vi "Main.vi"() -> ()   [LabVIEW 2016]
uses:
  <vilib>/picture/picture.llb/imagedata.ctl
panel:
  in  "Path":path
  in  "pConvertInfo In 2":T1
  out "QuitFlag":bool
  in  "image data":T2 caption="图像数据"
  in  "Rectangle":T3
  in  "pConvertInfo In":T1
  out "Picture":picture
  out "Acquired Frames/s":dbl
  out "Processed Frames/s":dbl
  in  "SavePic":bool
  in  "TriggerSource":u16(ring) items=["Software", "Line1", "Line2"]
  in  "ExecuteSoftTrig":bool
  in  "CloseTrig":bool
  in  "OpenTrig":bool
  in  "Stop":bool
  in  "Play":bool
  in  "Quit":bool
  in  "handle":i64
  in  "Height":i64
  in  "Width":i64
  in  "ExposureAuto":u16(ring) items=["Off", "Once", "Continuous"]
  in  "PixelFormat":u16(ring) items=["BayerRG8", "BayerGB8", "BayerRG10", "BayerGB10", "BayerRG10Packed", "BayerGB10Packed"]
  in  "GainRaw":dbl
  in  "ExposureTime":dbl
  in  "Close":bool
  in  "Open":bool
  out "IsGrabbing":bool
  out "HasDevices":bool
  out "TrigModeOn":bool
  in  "DeviceOpened":bool
  in  "DeviceList":u16(ring)
  out "error out":errorcluster
  in  "Discovery":bool
  in  "error in":errorcluster
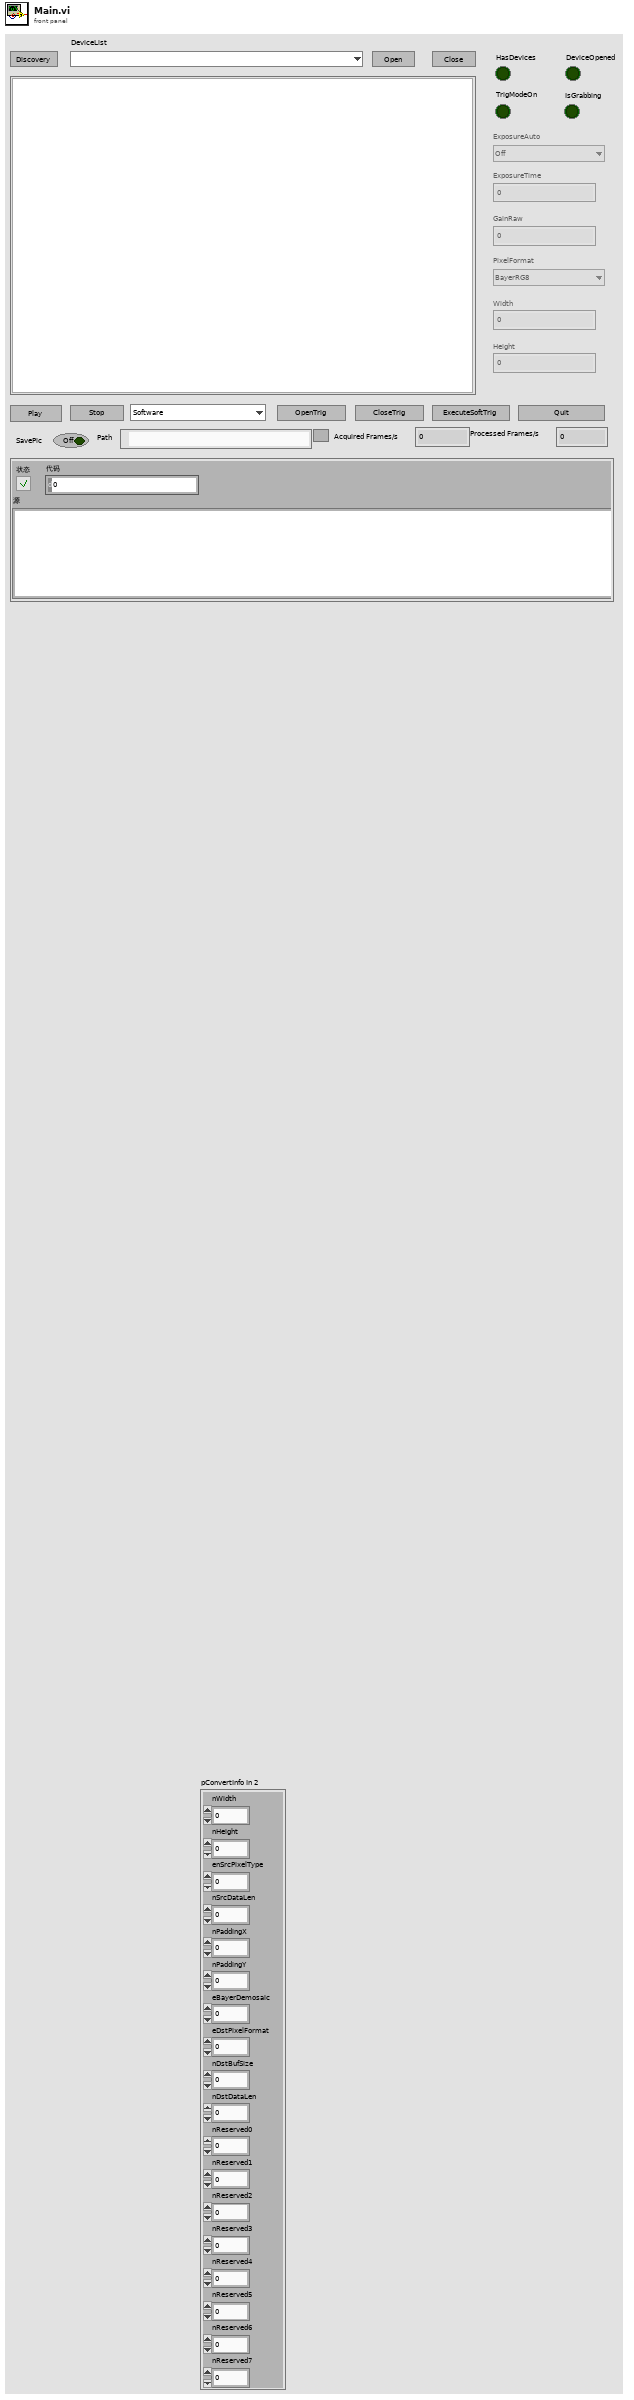
[diagram p1: front panel]
types:
  T1 = cluster{"nWidth":u32, "nHeight":u32, "enSrcPixelType":u32, "nSrcDataLen":u32, "nPaddingX":u32, "nPaddingY":u32, "eBayerDemosaic":u32, "eDstPixelFormat":u32, "nDstBufSize":u32, "nDstDataLen":u32, "nReserved0":u32, "nReserved1":u32, "nReserved2":u32, "nReserved3":u32, "nReserved4":u32, "nReserved5":u32, "nReserved6":u32, "nReserved7":u32}
  T2 = typedef "imagedata.ctl" = cluster{"image type":i32, "image depth":i32, "image":u8[], "mask":u8[], "colors":u32[], "Rectangle":cluster{"left":i16, "top":i16, "right":i16, "bottom":i16}}
  T3 = cluster{"left":i16, "top":i16, "right":i16, "bottom":i16}
  T4 = enum8{"Enabled", "Disabled", "Disabled and Grayed Out"}
  T5 = cluster{"blockId":u64, "status":u32, "width":u32, "height":u32, "size":u32, "pixelFormat":u32, "timeStamp":u64, "chunkCount":u32, "paddingX":u32, "paddingY":u32, "recvFrameTime":u32}
  T6 = cluster{"blockId":u64, "status":u32, "width":u32, "height":u32, "size":u32, "pixelFormat":i32, "timeStamp":u64, "chunkCount":u32, "paddingX":u32, "paddingY":u32, "recvFrameTime":u32}
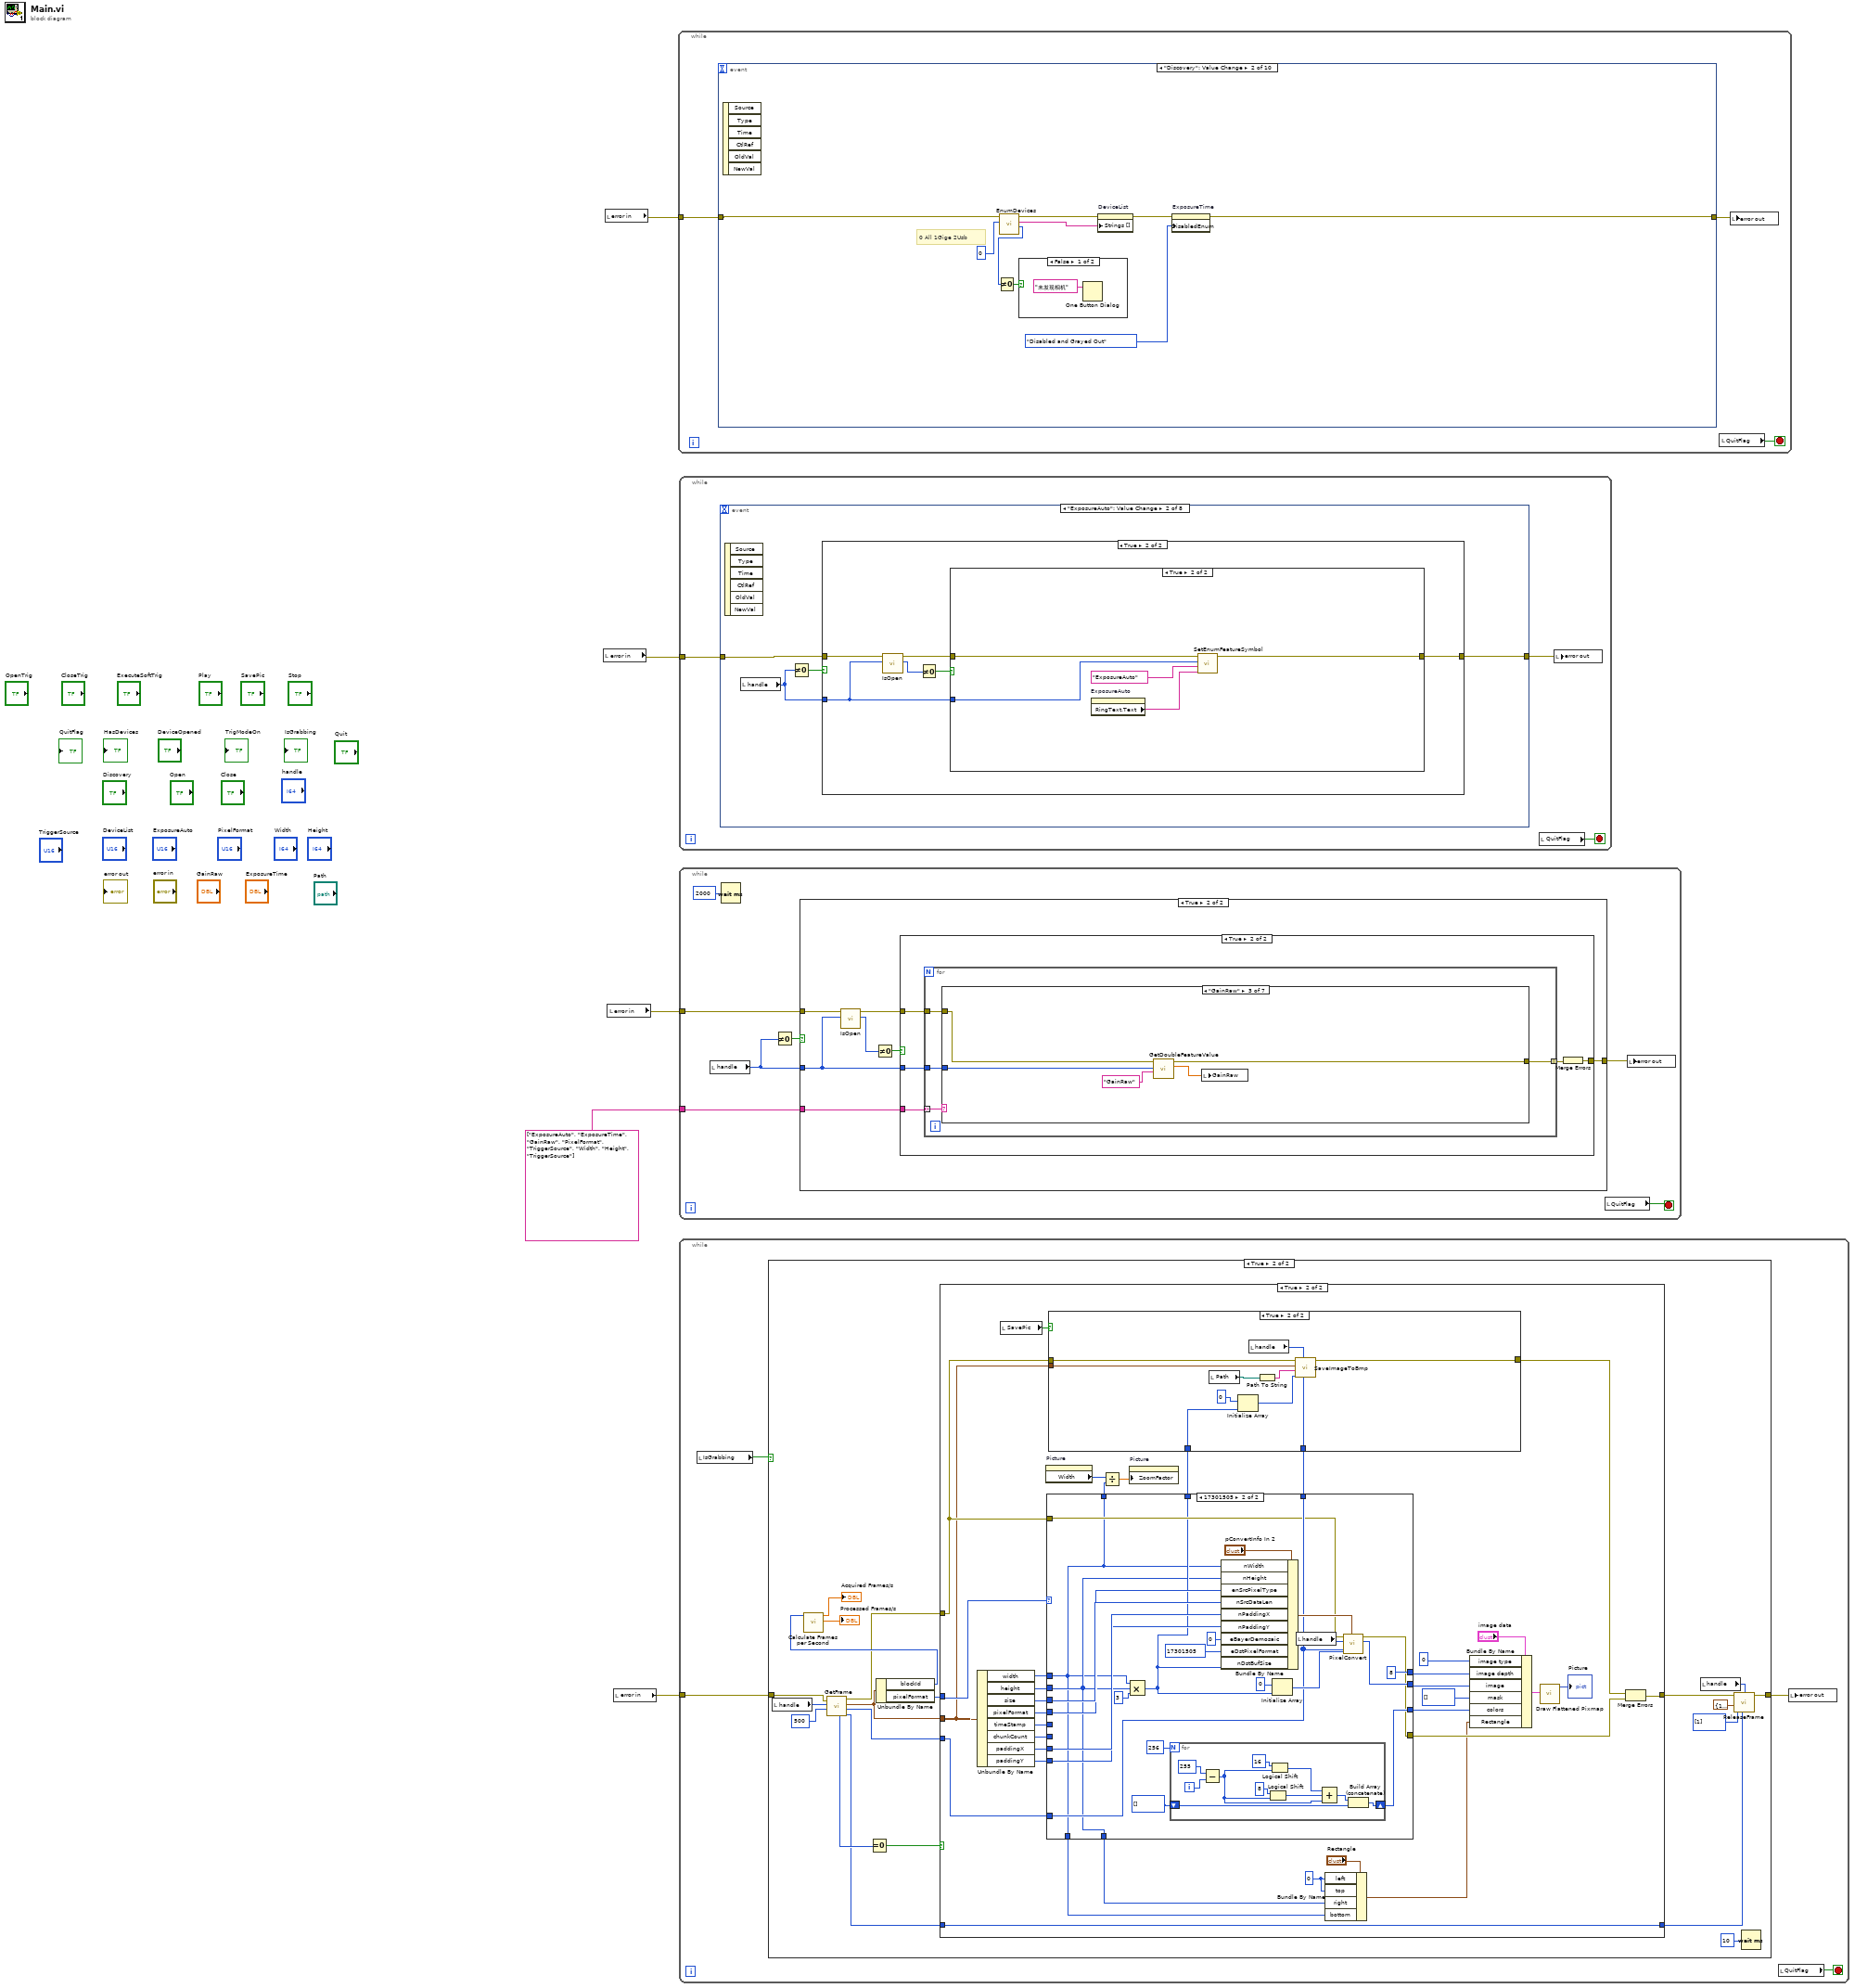
[diagram p0: block diagram]
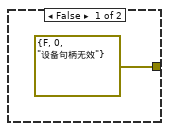
[diagram p2: hidden frame]
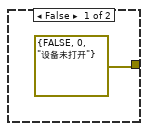
[diagram p3: hidden frame]
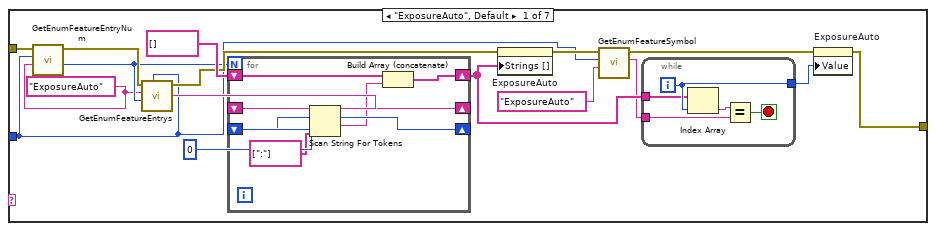
[diagram p4: hidden frame]
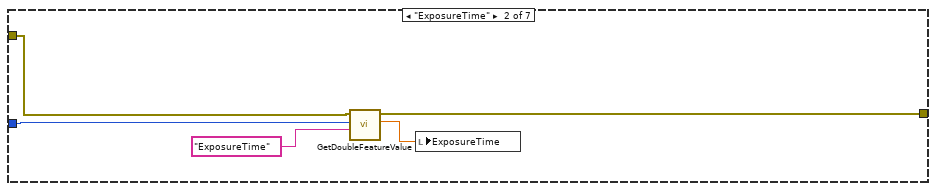
[diagram p5: hidden frame]
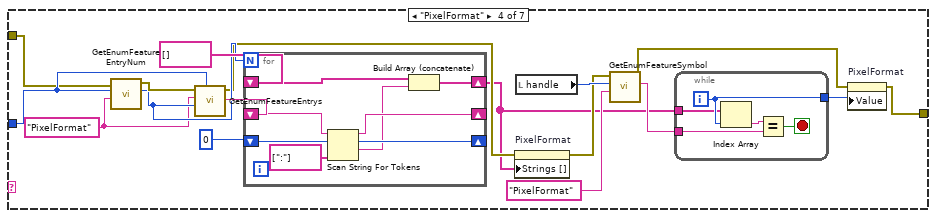
[diagram p6: hidden frame]
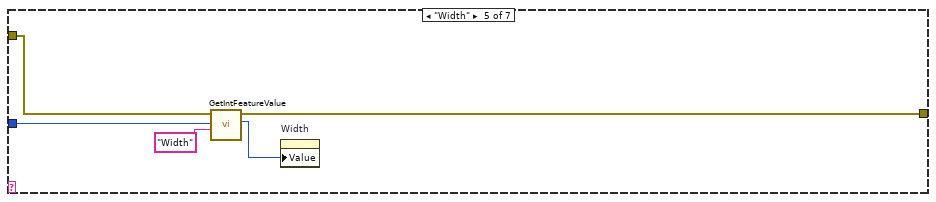
[diagram p7: hidden frame]
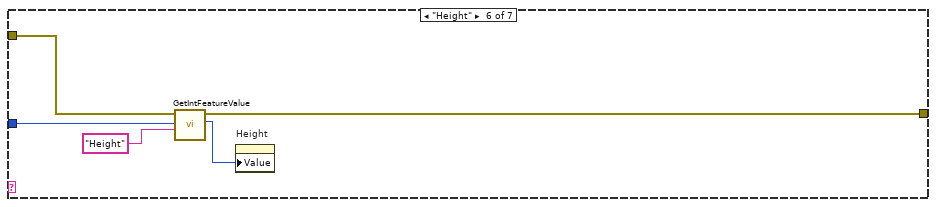
[diagram p8: hidden frame]
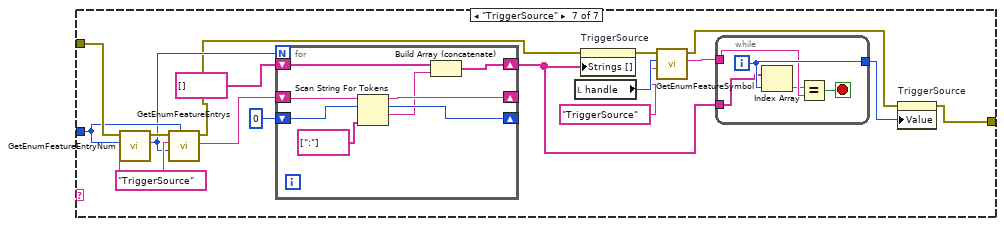
[diagram p9: hidden frame]
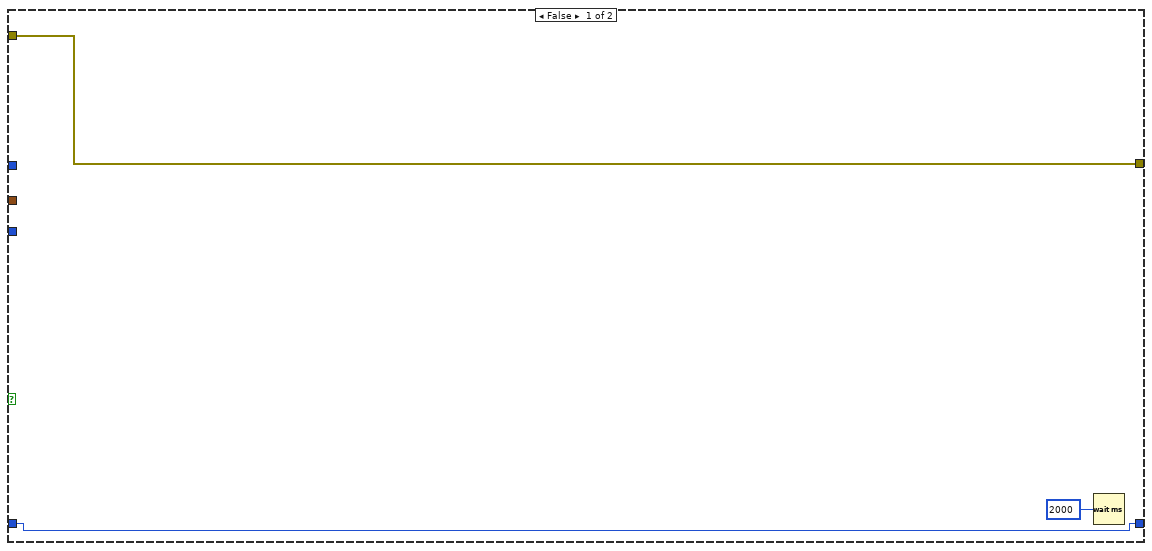
[diagram p11: hidden frame]
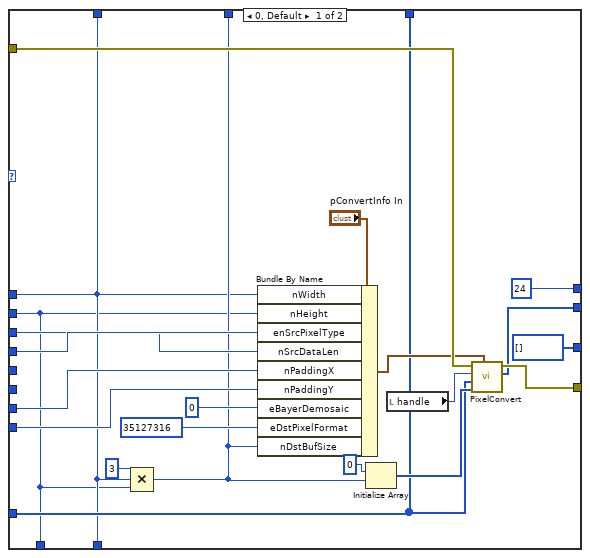
[diagram p13: hidden frame]
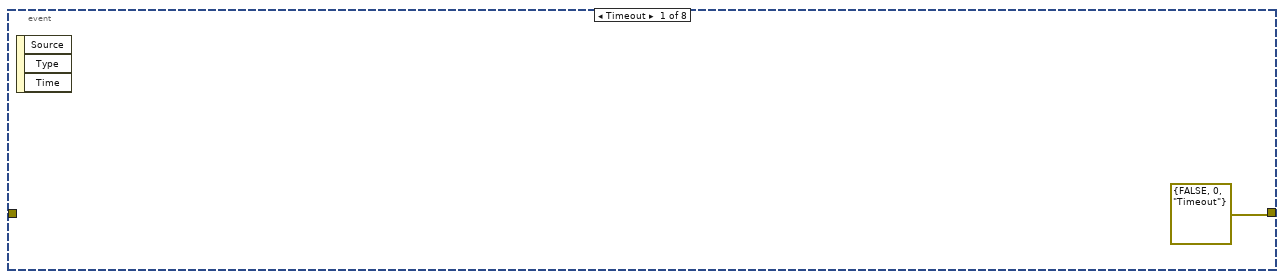
[diagram p14: hidden frame]
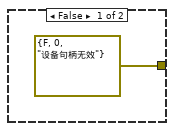
[diagram p15: hidden frame]
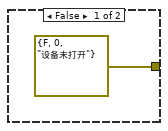
[diagram p16: hidden frame]
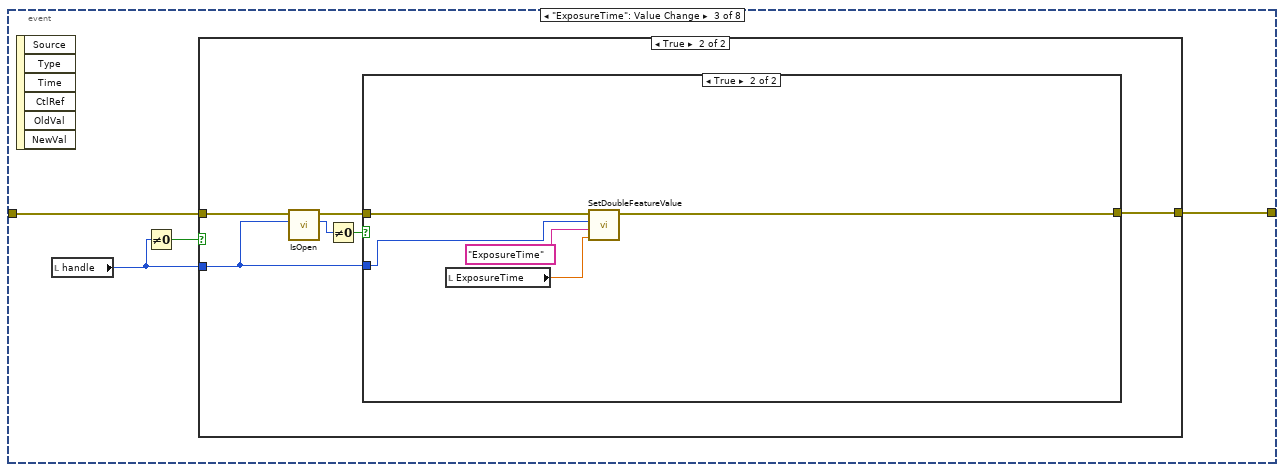
[diagram p17: hidden frame]
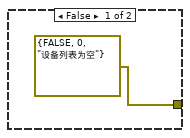
[diagram p18: hidden frame]
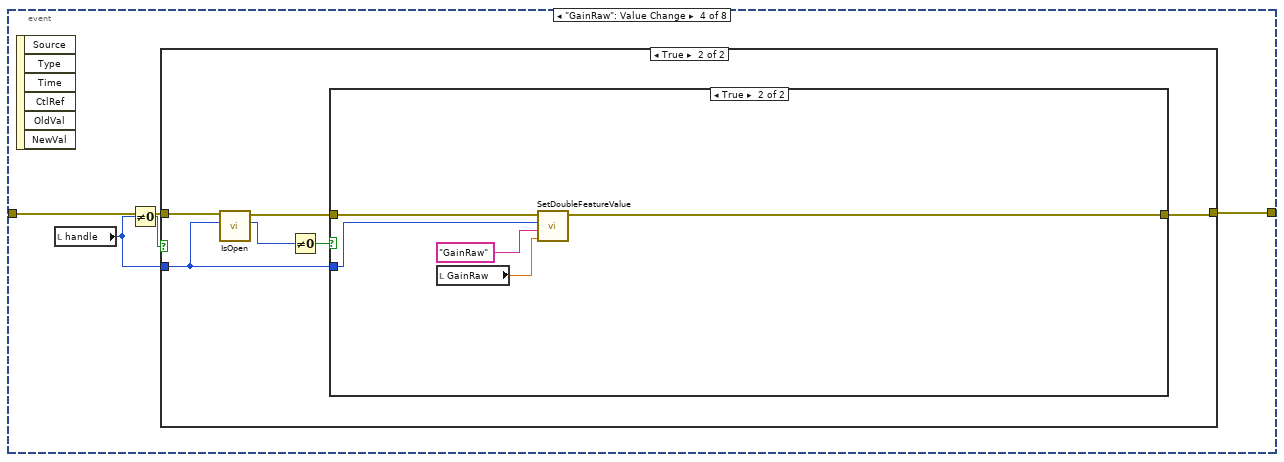
[diagram p20: hidden frame]
diagram:
  n1 = local read "error in"() -> (w4:errorcluster)
  n2 = local read "error in"() -> (w5:errorcluster)
  n3 = local read "error in"() -> (w2:errorcluster)
  n4 = local read "error in"() -> (w1:errorcluster)
  n5 = while {
    tunnel: w5 -> [w8]
    stop <- w7 stop-if-true
    n6 = event shown="[1] \"Discovery\": Value Change" {
      selector: _ -> [_ _ _ _ _ _ _ _ _ _]
      dyn-events: _ -> [_ _ _ _ _ _ _ _ _ _]
      timeout: _ -> [_ _ _ _ _ _ _ _ _ _]
      tunnel: w8 -> [_ w17 w23 w74 w87 w140 w147 w151 w169 w188]
      tunnel: [errorcluster {FALSE, 0, "Timeout"} w13 w22 w61 w85 w131 w143 w150 w155 w173] -> w6
      event Timeout {
        n7 = event-data() -> ()  [unwired: 1 in, 3 out]
      }
      event "Discovery": Value Change {
        # "0 All 1Gige 2Usb"
        n8 = event-data() -> ()  [unwired: 1 in, 6 out]
        n9 = call "EnumDevices.vi"("interfaceType"=u32 0, "error in"=w17) -> ("nDevNum"=w10:i32, "cameraKeyList"=w15:string[], "error out"=w16:errorcluster)  [unwired: 7 in]
        n10 = Not Equal To 0?(x=w10) -> (x != 0?=w11:bool)
        n11 = case shown="False" w11 {
          frame False {
            n12 = One Button Dialog(message="未发现相机") -> ()  [unwired: 1 in, 1 out]
          }
          frame True {
            n13 = local write "HasDevices"(TRUE ("HasDevices")) -> ()
          }
        }
        n14 = property on="DeviceList" class="Ring (strict)"(error in=w16, "Strings []"=w15) -> (error out=w12:errorcluster)  [unwired: 1 in, 1 out]
        n15 = property on="ExposureTime" class="DigNum (strict)"(error in=w12, "DisabledEnum"=T4."Disabled and Grayed Out" ("Disabled")) -> (error out=w13:errorcluster)  [unwired: 1 in, 1 out]
      }
      event "Quit": Value Change {
        n16 = event-data() -> ()  [unwired: 1 in, 6 out]
        n17 = flat-sequence {
          tunnel: w23 -> [w26]
          tunnel: [w26] -> w21
          tunnel: [w35] -> w22
          tunnel: w21 -> [w53]
          frame #0 {
            n18 = local write "SavePic"(FALSE ("SavePic")) -> ()
            n19 = Wait (ms)(milliseconds to wait=u32 500) -> ()  [unwired: 1 out]
          }
          frame #1 {
            (unwired) T4."Enabled" ("Disabled")
            (unwired) T4."Disabled and Grayed Out" ("Disabled")
            n20 = local read "handle"() -> (w29:i64)
            n21 = call "SetEnumFeatureSymbol.vi"("pEnumSymbol"="Off", "pFeatureName"="TriggerMode", "handle"=w29, "error in (no error)"=w53) -> ("return type"=w50:i32, "error out"=w48:errorcluster)  [unwired: 6 in]
            n22 = Equal To 0?(x=w50) -> (x = 0?=w49:bool)
            n23 = case shown="True" w49 {
              frame False {
              }
              frame True {
                n24 = local write "TrigModeOn"(FALSE ("IsGrabbing")) -> ()
              }
            }
            n25 = call "StopGrabbing.vi"("handle"=w29, "error in (no error)"=w48) -> ("return type"=w28:i32, "error out"=w36:errorcluster)  [unwired: 8 in]
            n26 = Equal To 0?(x=w28) -> (x = 0?=w27:bool)
            n27 = case shown="True" w27 {
              frame False {
              }
              frame True {
                n28 = local write "IsGrabbing"(FALSE ("IsGrabbing")) -> ()
              }
            }
            n29 = property on="ExposureAuto" class="Ring (strict)"(error in=w36, "DisabledEnum"=T4."Disabled and Grayed Out" ("Disabled")) -> (error out=w39:errorcluster)  [unwired: 1 in, 1 out]
            n30 = property on="GainRaw" class="DigNum (strict)"(error in=w39, "DisabledEnum"=T4."Disabled and Grayed Out" ("Disabled")) -> (error out=w37:errorcluster)  [unwired: 1 in, 1 out]
            n31 = property on="Height" class="DigNum (strict)"(error in=w37, "DisabledEnum"=T4."Disabled and Grayed Out" ("Disabled")) -> (error out=w45:errorcluster)  [unwired: 1 in, 1 out]
            n32 = property on="PixelFormat" class="Ring (strict)"(error in=w45, "DisabledEnum"=T4."Disabled and Grayed Out" ("Disabled")) -> (error out=w40:errorcluster)  [unwired: 1 in, 1 out]
            n33 = property on="ExposureTime" class="DigNum (strict)"(error in=w40, "DisabledEnum"=T4."Disabled and Grayed Out" ("Disabled")) -> (error out=w46:errorcluster)  [unwired: 1 in, 1 out]
            n34 = property on="Width" class="DigNum (strict)"(error in=w46, "DisabledEnum"=T4."Disabled and Grayed Out" ("Disabled")) -> (error out=w30:errorcluster)  [unwired: 1 in, 1 out]
            n35 = call "Close.vi"("handle"=w29, "error in (no error)"=w30) -> ("return type"=w33:i32, "error out"=w35:errorcluster)  [unwired: 8 in]
            n36 = Equal To 0?(x=w33) -> (x = 0?=w34:bool)
            n37 = case shown="True" w34 {
              frame False {
              }
              frame True {
                n38 = local write "DeviceOpened"(FALSE ("DeviceOpened")) -> ()
              }
            }
            n39 = local write "HasDevices"(FALSE ("HasDevices")) -> ()
            n40 = local write "QuitFlag"(FALSE) -> ()
            n41 = property on="DeviceList" class="Ring (strict)"("Strings []"=string[] []) -> ()  [unwired: 2 in, 2 out]
          }
        }
      }
      event "Open": Value Change {
        (unwired) T4."Enabled" ("Disabled")
        n42 = event-data() -> ()  [unwired: 1 in, 6 out]
        n43 = property on="DeviceList" class="Ring (strict)"(error in=w74) -> (error out=w76:errorcluster, "Value"=w75:u16)  [unwired: 1 in, 1 out]
        n44 = call "OpenDevice.vi"("pIdentifier"=w75, "error in (no error)"=w76) -> ("handle"=w60:i64, "retrun type"=w58:i32, "error out"=w62:errorcluster)  [unwired: 7 in]
        n45 = local write "handle"(w60) -> ()
        n46 = Equal To 0?(x=w58) -> (x = 0?=w59:bool)
        n47 = case shown="True" w59 {
          tunnel: w58 -> [w79 _]
          frame False {
            n48 = Number To Decimal String(number=w79) -> (decimal integer string=w78:string)  [unwired: 1 in]
            n49 = Concatenate Strings("打开相机失败" ("string"), w78) -> (w80:string)
            n50 = One Button Dialog(message=w80) -> ()  [unwired: 1 in, 1 out]
          }
          frame True {
            n51 = local write "DeviceOpened"(TRUE ("DeviceOpened")) -> ()
          }
        }
        n52 = property on="ExposureAuto" class="Ring (strict)"(error in=w62, "DisabledEnum"=T4."Enabled" ("Disabled")) -> (error out=w65:errorcluster)  [unwired: 1 in, 1 out]
        n53 = property on="GainRaw" class="DigNum (strict)"(error in=w65, "DisabledEnum"=T4."Enabled" ("Disabled")) -> (error out=w63:errorcluster)  [unwired: 1 in, 1 out]
        n54 = property on="Height" class="DigNum (strict)"(error in=w63, "DisabledEnum"=T4."Enabled" ("Disabled")) -> (error out=w71:errorcluster)  [unwired: 1 in, 1 out]
        n55 = property on="PixelFormat" class="Ring (strict)"(error in=w71, "DisabledEnum"=T4."Enabled" ("Disabled")) -> (error out=w66:errorcluster)  [unwired: 1 in, 1 out]
        n56 = property on="ExposureTime" class="DigNum (strict)"(error in=w66, "DisabledEnum"=T4."Enabled" ("Disabled")) -> (error out=w72:errorcluster)  [unwired: 1 in, 1 out]
        n57 = property on="Width" class="DigNum (strict)"(error in=w72, "DisabledEnum"=T4."Enabled" ("Disabled")) -> (error out=w61:errorcluster)  [unwired: 1 in, 1 out]
      }
      event "Play": Value Change {
        n58 = event-data() -> ()  [unwired: 1 in, 6 out]
        n59 = property on="DeviceList" class="Ring (strict)"(error in=w87) -> (error out=w86:errorcluster, "NumItems"=w83:u32)  [unwired: 1 in, 1 out]
        n60 = local read "handle"() -> (w82:i64)
        n61 = Not Equal To 0?(x=w83) -> (x != 0?=w84:bool)
        n62 = case shown="True" w84 {
          tunnel: w86 -> [_ w93]
          tunnel: [errorcluster {FALSE, 0, "设备列表为空"} w94] -> w85
          tunnel: w82 -> [_ w91]
          frame False {
          }
          frame True {
            n63 = call "IsOpen.vi"("handle"=w91, "error in (no error)"=w93) -> ("return type"=w89:i8, "error out"=w92:errorcluster)  [unwired: 8 in]
            n64 = Not Equal To 0?(x=w89) -> (x != 0?=w90:bool)
            n65 = case shown="True" w90 {
              tunnel: [w95 w101] -> w94
              tunnel: w91 -> [_ w99]
              tunnel: w92 -> [w95 w96]
              frame False {
              }
              frame True {
                n66 = call "IsGrabbing.vi"("handle"=w99, "error in (no error)"=w96) -> ("return type"=w97:i8, "error out"=w100:errorcluster)  [unwired: 8 in]
                n67 = Equal To 0?(x=w97) -> (x = 0?=w98:bool)
                n68 = case shown="True" w98 {
                  tunnel: [w102 w109] -> w101
                  tunnel: w100 -> [w102 w107]
                  tunnel: w99 -> [_ w106]
                  frame False {
                  }
                  frame True {
                    n69 = call "StartGrabbing.vi"("handle"=w106, "error in (no error)"=w107) -> ("retrun type"=w103:i32, "error out"=w105:errorcluster)  [unwired: 8 in]
                    n70 = Equal To 0?(x=w103) -> (x = 0?=w104:bool)
                    n71 = case shown="False" w104 {
                      frame False {
                        n72 = One Button Dialog(message="开始拉流失败") -> ()  [unwired: 1 in, 1 out]
                      }
                      frame True {
                        n73 = local write "IsGrabbing"(TRUE ("IsGrabbing")) -> ()
                      }
                    }
                    n74 = property on="ExposureAuto" class="Ring (strict)"(error in=w105, "DisabledEnum"=T4."Enabled" ("Disabled")) -> (error out=w118:errorcluster)  [unwired: 1 in, 1 out]
                    n75 = property on="Width" class="DigNum (strict)"(error in=w118, "DisabledEnum"=T4."Disabled and Grayed Out" ("Disabled")) -> (error out=w116:errorcluster)  [unwired: 1 in, 1 out]
                    n76 = property on="Height" class="DigNum (strict)"(error in=w116, "DisabledEnum"=T4."Disabled and Grayed Out" ("Disabled")) -> (error out=w115:errorcluster)  [unwired: 1 in, 1 out]
                    n77 = property on="GainRaw" class="DigNum (strict)"(error in=w115, "DisabledEnum"=T4."Enabled" ("Disabled")) -> (error out=w114:errorcluster)  [unwired: 1 in, 1 out]
                    n78 = property on="PixelFormat" class="Ring (strict)"(error in=w114, "DisabledEnum"=T4."Disabled and Grayed Out" ("Disabled")) -> (error out=w110:errorcluster)  [unwired: 1 in, 1 out]
                    n79 = property on="ExposureTime" class="DigNum (strict)"(error in=w110, "DisabledEnum"=T4."Enabled" ("Disabled")) -> (error out=w109:errorcluster)  [unwired: 1 in, 1 out]
                  }
                }
              }
            }
          }
        }
      }
      event "OpenTrig": Value Change {
        n80 = event-data() -> ()  [unwired: 1 in, 6 out]
        n81 = local read "handle"() -> (w137:i64)
        n82 = property on="TriggerSource" class="Ring (strict)"() -> ("RingText.Text"=w127:string)  [unwired: 2 in, 2 out]
        n83 = call "SetEnumFeatureSymbol.vi"("pEnumSymbol"=w127, "pFeatureName"="TriggerSource", "handle"=w137, "error in (no error)"=w140) -> ("return type"=w129:i32, "error out"=w139:errorcluster)  [unwired: 6 in]
        n84 = Equal To 0?(x=w129) -> (x = 0?=w126:bool)
        n85 = call "SetEnumFeatureSymbol.vi"("pEnumSymbol"="FrameStart", "pFeatureName"="TriggerSelector", "handle"=w137, "error in (no error)"=w139) -> ("return type"=w128:i32, "error out"=w138:errorcluster)  [unwired: 6 in]
        n86 = Equal To 0?(x=w128) -> (x = 0?=w125:bool)
        n87 = And(x=w125, y=w126) -> (x .and. y?=w124:bool)
        n88 = call "SetEnumFeatureSymbol.vi"("pEnumSymbol"="On", "pFeatureName"="TriggerMode", "handle"=w137, "error in (no error)"=w138) -> ("return type"=w130:i32, "error out"=w131:errorcluster)  [unwired: 6 in]
        n89 = Equal To 0?(x=w130) -> (x = 0?=w123:bool)
        n90 = And(x=w123, y=w124) -> (x .and. y?=w122:bool)
        n91 = local write "TrigModeOn"(w122) -> ()
      }
      event "CloseTrig": Value Change {
        n92 = event-data() -> ()  [unwired: 1 in, 6 out]
        n93 = local read "handle"() -> (w146:i64)
        n94 = call "SetEnumFeatureSymbol.vi"("pEnumSymbol"="Off", "pFeatureName"="TriggerMode", "handle"=w146, "error in (no error)"=w147) -> ("return type"=w142:i32, "error out"=w143:errorcluster)  [unwired: 6 in]
        n95 = Equal To 0?(x=w142) -> (x = 0?=w141:bool)
        n96 = case shown="True" w141 {
          frame False {
          }
          frame True {
            n97 = local write "TrigModeOn"(FALSE ("TrigModeOn")) -> ()
          }
        }
      }
      event "ExecuteSoftTrig": Value Change {
        n98 = event-data() -> ()  [unwired: 1 in, 6 out]
        n99 = local read "handle"() -> (w149:i64)
        n100 = call "ExecuteCommandFeature.vi"("pFeatureName"="TriggerSoftware", "handle"=w149, "error in (no error)"=w151) -> ("error out"=w150:errorcluster)  [unwired: 8 in]
      }
      event "Stop": Value Change {
        n101 = event-data() -> ()  [unwired: 1 in, 6 out]
        n102 = local read "handle"() -> (w168:i64)
        n103 = call "StopGrabbing.vi"("handle"=w168, "error in (no error)"=w169) -> ("return type"=w153:i32, "error out"=w162:errorcluster)  [unwired: 8 in]
        n104 = Equal To 0?(x=w153) -> (x = 0?=w154:bool)
        n105 = case shown="True" w154 {
          frame False {
          }
          frame True {
            n106 = local write "IsGrabbing"(FALSE ("IsGrabbing")) -> ()
          }
        }
        n107 = property on="ExposureAuto" class="Ring (strict)"(error in=w162, "DisabledEnum"=T4."Enabled" ("Disabled")) -> (error out=w163:errorcluster)  [unwired: 1 in, 1 out]
        n108 = property on="ExposureTime" class="DigNum (strict)"(error in=w163, "DisabledEnum"=T4."Enabled" ("Disabled")) -> (error out=w164:errorcluster)  [unwired: 1 in, 1 out]
        n109 = property on="GainRaw" class="DigNum (strict)"(error in=w164, "DisabledEnum"=T4."Enabled" ("Disabled")) -> (error out=w165:errorcluster)  [unwired: 1 in, 1 out]
        n110 = property on="Width" class="DigNum (strict)"(error in=w165, "DisabledEnum"=T4."Enabled" ("Disabled")) -> (error out=w166:errorcluster)  [unwired: 1 in, 1 out]
        n111 = property on="Height" class="DigNum (strict)"(error in=w166, "DisabledEnum"=T4."Enabled" ("Disabled")) -> (error out=w167:errorcluster)  [unwired: 1 in, 1 out]
        n112 = property on="PixelFormat" class="Ring (strict)"(error in=w167, "DisabledEnum"=T4."Enabled" ("Disabled")) -> (error out=w155:errorcluster)  [unwired: 1 in, 1 out]
      }
      event "Close": Value Change {
        (unwired) T4."Disabled and Grayed Out" ("Disabled")
        n113 = event-data() -> ()  [unwired: 1 in, 6 out]
        n114 = property on="handle" class="DigNum (strict)"(error in=w188) -> (error out=w187:errorcluster, "Value"=w186:i64)  [unwired: 1 in, 1 out]
        n115 = call "Close.vi"("handle"=w186, "error in (no error)"=w187) -> ("return type"=w172:i32, "error out"=w174:errorcluster)  [unwired: 8 in]
        n116 = Equal To 0?(x=w172) -> (x = 0?=w171:bool)
        n117 = case shown="True" w171 {
          frame False {
          }
          frame True {
            n118 = local write "DeviceOpened"(FALSE ("DeviceOpened")) -> ()
          }
        }
        n119 = property on="GainRaw" class="DigNum (strict)"(error in=w174, "DisabledEnum"=T4."Disabled and Grayed Out" ("Disabled")) -> (error out=w177:errorcluster)  [unwired: 1 in, 1 out]
        n120 = property on="Height" class="DigNum (strict)"(error in=w177, "DisabledEnum"=T4."Disabled and Grayed Out" ("Disabled")) -> (error out=w175:errorcluster)  [unwired: 1 in, 1 out]
        n121 = property on="Width" class="DigNum (strict)"(error in=w175, "DisabledEnum"=T4."Disabled and Grayed Out" ("Disabled")) -> (error out=w183:errorcluster)  [unwired: 1 in, 1 out]
        n122 = property on="ExposureTime" class="DigNum (strict)"(error in=w183, "DisabledEnum"=T4."Disabled and Grayed Out" ("Disabled")) -> (error out=w178:errorcluster)  [unwired: 1 in, 1 out]
        n123 = property on="ExposureAuto" class="Ring (strict)"(error in=w178, "DisabledEnum"=T4."Disabled and Grayed Out" ("Disabled")) -> (error out=w184:errorcluster)  [unwired: 1 in, 1 out]
        n124 = property on="PixelFormat" class="Ring (strict)"(error in=w184, "DisabledEnum"=T4."Disabled and Grayed Out" ("Disabled")) -> (error out=w173:errorcluster)  [unwired: 1 in, 1 out]
      }
    }
    n125 = local read "QuitFlag"() -> (w7:bool)
    n126 = local write "error out"(w6) -> ()
  }
  n127 = while {
    tunnel: w4 -> [w192]
    stop <- w190 stop-if-true
    n128 = event shown="[1] \"ExposureAuto\": Value Change" {
      selector: _ -> [_ _ _ _ _ _ _ _]
      dyn-events: _ -> [_ _ _ _ _ _ _ _]
      timeout: _ -> [_ _ _ _ _ _ _ _]
      tunnel: [errorcluster {FALSE, 0, "Timeout"} w197 w214 w231 w248 w265 w282 w298] -> w191
      tunnel: w192 -> [_ w194 w213 w230 w247 w264 w281 w297]
      event Timeout {
        n129 = event-data() -> ()  [unwired: 1 in, 3 out]
      }
      event "ExposureAuto": Value Change {
        n130 = event-data() -> ()  [unwired: 1 in, 6 out]
        n131 = local read "handle"() -> (w195:i64)
        n132 = Not Equal To 0?(x=w195) -> (x != 0?=w196:bool)
        n133 = case shown="True" w196 {
          tunnel: [errorcluster {"status"=FALSE, "code"=0, "source"="设备句柄无效"} ("错误常量") w203] -> w197
          tunnel: w195 -> [_ w201]
          tunnel: w194 -> [_ w202]
          frame False {
          }
          frame True {
            n134 = call "IsOpen.vi"("handle"=w201, "error in (no error)"=w202) -> ("return type"=w199:i8, "error out"=w204:errorcluster)  [unwired: 8 in]
            n135 = Not Equal To 0?(x=w199) -> (x != 0?=w200:bool)
            n136 = case shown="True" w200 {
              tunnel: w204 -> [_ w208]
              tunnel: [errorcluster {"status"=FALSE, "code"=0, "source"="设备未打开"} ("错误常量") w207] -> w203
              tunnel: w201 -> [_ w206]
              frame False {
              }
              frame True {
                n137 = property on="ExposureAuto" class="Ring (strict)"() -> ("RingText.Text"=w209:string)  [unwired: 2 in, 2 out]
                n138 = call "SetEnumFeatureSymbol.vi"("pEnumSymbol"=w209, "pFeatureName"="ExposureAuto", "handle"=w206, "error in (no error)"=w208) -> ("error out"=w207:errorcluster)  [unwired: 6 in, 1 out]
              }
            }
          }
        }
      }
      event "ExposureTime": Value Change {
        n139 = event-data() -> ()  [unwired: 1 in, 6 out]
        n140 = local read "handle"() -> (w212:i64)
        n141 = Not Equal To 0?(x=w212) -> (x != 0?=w211:bool)
        n142 = case shown="True" w211 {
          tunnel: [errorcluster {FALSE, 0, "设备列表为空"} w220] -> w214
          tunnel: w213 -> [_ w219]
          tunnel: w212 -> [_ w218]
          frame False {
          }
          frame True {
            n143 = call "IsOpen.vi"("handle"=w218, "error in (no error)"=w219) -> ("return type"=w217:i8, "error out"=w221:errorcluster)  [unwired: 8 in]
            n144 = Not Equal To 0?(x=w217) -> (x != 0?=w216:bool)
            n145 = case shown="True" w216 {
              tunnel: w221 -> [w222 w227]
              tunnel: [w222 w224] -> w220
              tunnel: w218 -> [_ w223]
              frame False {
              }
              frame True {
                n146 = local read "ExposureTime"() -> (w225:dbl)
                n147 = call "SetDoubleFeatureValue.vi"("doubleValue"=w225, "pFeatureName"="ExposureTime", "handle"=w223, "error in (no error)"=w227) -> ("error out"=w224:errorcluster)  [unwired: 7 in]
              }
            }
          }
        }
      }
      event "GainRaw": Value Change {
        n148 = event-data() -> ()  [unwired: 1 in, 6 out]
        n149 = local read "handle"() -> (w228:i64)
        n150 = Not Equal To 0?(x=w228) -> (x != 0?=w229:bool)
        n151 = case shown="True" w229 {
          tunnel: [errorcluster {FALSE, 0, "设备句柄无效"} w237] -> w231
          tunnel: w230 -> [_ w236]
          tunnel: w228 -> [_ w235]
          frame False {
          }
          frame True {
            n152 = call "IsOpen.vi"("handle"=w235, "error in (no error)"=w236) -> ("return type"=w233:i8, "error out"=w238:errorcluster)  [unwired: 8 in]
            n153 = Not Equal To 0?(x=w233) -> (x != 0?=w234:bool)
            n154 = case shown="True" w234 {
              tunnel: [errorcluster {FALSE, 0, "设备未打开"} w243] -> w237
              tunnel: w238 -> [_ w244]
              tunnel: w235 -> [_ w240]
              frame False {
              }
              frame True {
                n155 = local read "GainRaw"() -> (w241:dbl)
                n156 = call "SetDoubleFeatureValue.vi"("doubleValue"=w241, "pFeatureName"="GainRaw", "handle"=w240, "error in (no error)"=w244) -> ("error out"=w243:errorcluster)  [unwired: 7 in]
              }
            }
          }
        }
      }
      event "PixelFormat": Value Change {
        n157 = event-data() -> ()  [unwired: 1 in, 6 out]
        n158 = local read "handle"() -> (w245:i64)
        n159 = Not Equal To 0?(x=w245) -> (x != 0?=w246:bool)
        n160 = case shown="True" w246 {
          tunnel: [errorcluster {FALSE, 0, "设备句柄无效"} w254] -> w248
          tunnel: w245 -> [_ w253]
          tunnel: w247 -> [_ w252]
          frame False {
          }
          frame True {
            n161 = call "IsOpen.vi"("handle"=w253, "error in (no error)"=w252) -> ("return type"=w250:i8, "error out"=w255:errorcluster)  [unwired: 8 in]
            n162 = Not Equal To 0?(x=w250) -> (x != 0?=w251:bool)
            n163 = case shown="True" w251 {
              tunnel: w255 -> [_ w261]
              tunnel: [errorcluster {FALSE, 0, "设备未打开"} w260] -> w254
              tunnel: w253 -> [_ w257]
              frame False {
              }
              frame True {
                n164 = property on="PixelFormat" class="Ring (strict)"() -> ("RingText.Text"=w258:string)  [unwired: 2 in, 2 out]
                n165 = call "SetEnumFeatureSymbol.vi"("pEnumSymbol"=w258, "pFeatureName"="PixelFormat", "handle"=w257, "error in (no error)"=w261) -> ("error out"=w260:errorcluster)  [unwired: 6 in, 1 out]
              }
            }
          }
        }
      }
      event "Width": Value Change {
        n166 = event-data() -> ()  [unwired: 1 in, 6 out]
        n167 = local read "handle"() -> (w262:i64)
        n168 = Not Equal To 0?(x=w262) -> (x != 0?=w263:bool)
        n169 = case shown="True" w263 {
          tunnel: [errorcluster {FALSE, 0, "设备句柄无效"} w271] -> w265
          tunnel: w264 -> [_ w270]
          tunnel: w262 -> [_ w269]
          frame False {
          }
          frame True {
            n170 = call "IsOpen.vi"("handle"=w269, "error in (no error)"=w270) -> ("return type"=w267:i8, "error out"=w272:errorcluster)  [unwired: 8 in]
            n171 = Not Equal To 0?(x=w267) -> (x != 0?=w268:bool)
            n172 = case shown="True" w268 {
              tunnel: w272 -> [_ w278]
              tunnel: [errorcluster {FALSE, 0, "设备未打开"} w275] -> w271
              tunnel: w269 -> [_ w274]
              frame False {
              }
              frame True {
                n173 = local read "Width"() -> (w276:i64)
                n174 = call "SetIntFeatureValue.vi"("intValue"=w276, "pFeatureName"="Width", "handle"=w274, "error in (no error)"=w278) -> ("error out"=w275:errorcluster)  [unwired: 7 in]
              }
            }
          }
        }
      }
      event "Height": Value Change {
        n175 = event-data() -> ()  [unwired: 1 in, 6 out]
        n176 = local read "handle"() -> (w279:i64)
        n177 = Not Equal To 0?(x=w279) -> (x != 0?=w280:bool)
        n178 = case shown="True" w280 {
          tunnel: [errorcluster {FALSE, 0, "设备句柄无效"} w288] -> w282
          tunnel: w281 -> [_ w287]
          tunnel: w279 -> [_ w286]
          frame False {
          }
          frame True {
            n179 = call "IsOpen.vi"("handle"=w286, "error in (no error)"=w287) -> ("return type"=w285:i8, "error out"=w289:errorcluster)  [unwired: 8 in]
            n180 = Not Equal To 0?(x=w285) -> (x != 0?=w284:bool)
            n181 = case shown="True" w284 {
              tunnel: w289 -> [_ w295]
              tunnel: [errorcluster {FALSE, 0, "设备未打开"} w294] -> w288
              tunnel: w286 -> [_ w291]
              frame False {
              }
              frame True {
                n182 = local read "Height"() -> (w292:i64)
                n183 = call "SetIntFeatureValue.vi"("intValue"=w292, "pFeatureName"="Height", "handle"=w291, "error in (no error)"=w295) -> ("error out"=w294:errorcluster)  [unwired: 7 in]
              }
            }
          }
        }
      }
      event "TriggerSource": Value Change {
        n184 = event-data() -> ()  [unwired: 1 in, 6 out]
        n185 = local read "handle"() -> (w296:i64)
        n186 = Not Equal To 0?(x=w296) -> (x != 0?=w299:bool)
        n187 = case shown="True" w299 {
          tunnel: [errorcluster {"status"=FALSE, "code"=0, "source"="设备句柄无效"} ("错误常量") w304] -> w298
          tunnel: w297 -> [_ w306]
          tunnel: w296 -> [_ w303]
          frame False {
          }
          frame True {
            n188 = call "IsOpen.vi"("handle"=w303, "error in (no error)"=w306) -> ("return type"=w301:i8, "error out"=w305:errorcluster)  [unwired: 8 in]
            n189 = Not Equal To 0?(x=w301) -> (x != 0?=w302:bool)
            n190 = case shown="True" w302 {
              tunnel: w305 -> [_ w321]
              tunnel: [errorcluster {"status"=FALSE, "code"=0, "source"="设备未打开"} ("错误常量") w317] -> w304
              tunnel: w303 -> [_ w310]
              frame False {
              }
              frame True {
                n191 = property on="TriggerSource" class="Ring (strict)"() -> ("RingText.Text"=w322:string)  [unwired: 2 in, 2 out]
                n192 = call "SetEnumFeatureSymbol.vi"("pEnumSymbol"=w322, "pFeatureName"="TriggerSource", "handle"=w310, "error in (no error)"=w321) -> ("error out"=w320:errorcluster)  [unwired: 6 in, 1 out]
                n193 = call "SetEnumFeatureSymbol.vi"("pEnumSymbol"="FrameStart", "pFeatureName"="TriggerSelector", "handle"=w310, "error in (no error)"=w320) -> ("error out"=w319:errorcluster)  [unwired: 6 in, 1 out]
                n194 = call "SetEnumFeatureSymbol.vi"("pEnumSymbol"="On", "pFeatureName"="TriggerMode", "handle"=w310, "error in (no error)"=w319) -> ("return type"=w308:i32, "error out"=w318:errorcluster)  [unwired: 6 in]
                n195 = Equal To 0?(x=w308) -> (x = 0?=w309:bool)
                n196 = case shown="True" w309 {
                  frame False {
                  }
                  frame True {
                    n197 = local write "TrigModeOn"(TRUE ("TrigModeOn")) -> ()
                  }
                }
                n198 = call "SetEnumFeatureSymbol.vi"("pEnumSymbol"="RisingEdge", "pFeatureName"="TriggerActivation", "handle"=w310, "error in (no error)"=w318) -> ("error out"=w317:errorcluster)  [unwired: 6 in, 1 out]
              }
            }
          }
        }
      }
    }
    n199 = local read "QuitFlag"() -> (w190:bool)
    n200 = local write "error out"(w191) -> ()
  }
  n201 = while {
    tunnel: string[] ["ExposureAuto", "ExposureTime", "GainRaw", "PixelFormat", "TriggerSource", "Width", "Height", "TriggerSource"] -> [w330]
    tunnel: w2 -> [w328]
    stop <- w325 stop-if-true
    n202 = local read "handle"() -> (w326:i64)
    n203 = Wait (ms)(milliseconds to wait=u32 2000) -> ()  [unwired: 1 out]
    n204 = Not Equal To 0?(x=w326) -> (x != 0?=w327:bool)
    n205 = case shown="True" w327 {
      tunnel: w330 -> [_ w339]
      tunnel: [errorcluster {"status"=FALSE, "code"=0, "source"="设备句柄无效"} ("错误常量") w337] -> w329
      tunnel: w328 -> [_ w336]
      tunnel: w326 -> [_ w335]
      frame False {
      }
      frame True {
        n206 = call "IsOpen.vi"("handle"=w335, "error in (no error)"=w336) -> ("return type"=w333:i8, "error out"=w338:errorcluster)  [unwired: 8 in]
        n207 = Not Equal To 0?(x=w333) -> (x != 0?=w334:bool)
        n208 = case shown="True" w334 {
          tunnel: w339 -> [_ w345]
          tunnel: w338 -> [_ w344]
          tunnel: [errorcluster {FALSE, 0, "设备未打开"} w343] -> w337
          tunnel: w335 -> [_ w341]
          frame False {
          }
          frame True {
            n209 = for {
              tunnel: w345 -> [w349] mode=indexing
              tunnel: w344 -> [w348]
              tunnel: [w347] -> w342 mode=indexing
              tunnel: w341 -> [w346]
              n210 = case shown="\"GainRaw\"" w349 {
                tunnel: w348 -> [w360 w381 w384 w393 w419 w427 w441]
                tunnel: [w361 w380 w386 w402 w422 w426 w429] -> w347
                tunnel: w346 -> [w353 w379 w385 w394 w420 w424 w434]
                frame "ExposureAuto", Default {
                  w354 = "ExposureAuto" ("pFeatureName")
                  n211 = call "GetEnumFeatureEntryNum.vi"("pFeatureName"=w354, "handle"=w353, "error in (no error)"=w360) -> ("pEntryNum"=w355:i64, "error out"=w365:errorcluster)  [unwired: 7 in]
                  n212 = call "GetEnumFeatureEntrys.vi"("handle"=w353, "EntryNum"=w355, "pFeatureName"=w354, "error in (no error)"=w365) -> ("pLbEnumEntryList out"=w362:string, "error out"=w358:errorcluster)  [unwired: 5 in, 1 out]
                  n213 = for {
                    N: w355 -> [_]
                    shift-right: [w376] -> _
                    shift-left: 0 ("offset") -> [w377]
                    shift-right: [w374] -> _
                    shift-left: w362 -> [w375]
                    shift-right: [w372] -> w352
                    shift-left: string[] [] -> [w373]
                    n214 = Scan String For Tokens(6:string[] [":"] ("delimiters (\\s,\\t,\\r,\\n)"), 8:w377, 9:w375) -> (1:w371:string, 2:w376:i32, 3:w374:string)  [unwired: 3 in, 1 out]
                    n215 = Build Array (concatenate)(w373, w371) -> (w372:string[])
                  }
                  n216 = property on="ExposureAuto" class="Ring (strict)"(error in=w358, "Strings []"=w352) -> (error out=w357:errorcluster)  [unwired: 1 in, 1 out]
                  n217 = call "GetEnumFeatureSymbol.vi"("pFeatureName"="ExposureAuto", "handle"=w353, "error in (no error)"=w357) -> ("pEnumSymbol"=w351:string, "error out"=w356:errorcluster)  [unwired: 7 in]
                  n218 = while {
                    tunnel: [w369] -> w350
                    tunnel: w352 -> [w368]
                    tunnel: w351 -> [w367]
                    i -> [w369]
                    stop <- w370 stop-if-true
                    n219 = Index Array(array=w368, index=w369) -> (element=w366:string)
                    n220 = Equal?(x=w366, y=w367) -> (x = y?=w370:bool)
                  }
                  n221 = property on="ExposureAuto" class="Ring (strict)"(error in=w356, "Value"=w350) -> (error out=w361:errorcluster)  [unwired: 1 in, 1 out]
                }
                frame "ExposureTime" {
                  n222 = call "GetDoubleFeatureValue.vi"("pFeatureName"="ExposureTime", "handle"=w379, "error in (no error)"=w381) -> ("pDoubleValue"=w382:dbl, "error out"=w380:errorcluster)  [unwired: 7 in]
                  n223 = local write "ExposureTime"(w382) -> ()
                }
                frame "GainRaw" {
                  n224 = call "GetDoubleFeatureValue.vi"("pFeatureName"="GainRaw", "handle"=w385, "error in (no error)"=w384) -> ("pDoubleValue"=w387:dbl, "error out"=w386:errorcluster)  [unwired: 7 in]
                  n225 = local write "GainRaw"(w387) -> ()
                }
                frame "PixelFormat" {
                  w392 = "PixelFormat" ("pFeatureName")
                  n226 = call "GetEnumFeatureEntryNum.vi"("pFeatureName"=w392, "handle"=w394, "error in (no error)"=w393) -> ("pEntryNum"=w400:i64, "error out"=w405:errorcluster)  [unwired: 7 in]
                  n227 = call "GetEnumFeatureEntrys.vi"("handle"=w394, "EntryNum"=w400, "pFeatureName"=w392, "error in (no error)"=w405) -> ("pLbEnumEntryList out"=w401:string, "error out"=w397:errorcluster)  [unwired: 5 in, 1 out]
                  n228 = for {
                    N: w400 -> [_]
                    shift-right: [w416] -> _
                    shift-left: 0 ("offset past token") -> [w417]
                    shift-right: [w414] -> _
                    shift-left: w401 -> [w415]
                    shift-right: [w412] -> w390
                    shift-left: string[] [] -> [w413]
                    n229 = Scan String For Tokens(6:string[] [":"] ("delimiters (\\s,\\t,\\r,\\n)"), 8:w417, 9:w415) -> (1:w411:string, 2:w416:i32, 3:w414:string)  [unwired: 3 in, 1 out]
                    n230 = Build Array (concatenate)(w413, w411) -> (w412:string[])
                  }
                  n231 = property on="PixelFormat" class="Ring (strict)"(error in=w397, "Strings []"=w390) -> (error out=w396:errorcluster)  [unwired: 1 in, 1 out]
                  n232 = local read "handle"() -> (w398:i64)
                  n233 = call "GetEnumFeatureSymbol.vi"("pFeatureName"="PixelFormat", "handle"=w398, "error in (no error)"=w396) -> ("pEnumSymbol"=w391:string, "error out"=w395:errorcluster)  [unwired: 7 in]
                  n234 = while {
                    tunnel: [w409] -> w389
                    tunnel: w390 -> [w408]
                    tunnel: w391 -> [w407]
                    i -> [w409]
                    stop <- w410 stop-if-true
                    n235 = Index Array(array=w408, index=w409) -> (element=w406:string)
                    n236 = Equal?(x=w406, y=w407) -> (x = y?=w410:bool)
                  }
                  n237 = property on="PixelFormat" class="Ring (strict)"(error in=w395, "Value"=w389) -> (error out=w402:errorcluster)  [unwired: 1 in, 1 out]
                }
                frame "Width" {
                  n238 = call "GetIntFeatureValue.vi"("pFeatureName"="Width", "handle"=w420, "error in (no error)"=w419) -> ("pIntValue"=w421:i64, "error out"=w422:errorcluster)  [unwired: 7 in]
                  n239 = property on="Width" class="DigNum (strict)"("Value"=w421) -> ()  [unwired: 2 in, 2 out]
                }
                frame "Height" {
                  n240 = call "GetIntFeatureValue.vi"("pFeatureName"="Height", "handle"=w424, "error in (no error)"=w427) -> ("pIntValue"=w425:i64, "error out"=w426:errorcluster)  [unwired: 7 in]
                  n241 = property on="Height" class="DigNum (strict)"("Value"=w425) -> ()  [unwired: 2 in, 2 out]
                }
                frame "TriggerSource" {
                  w440 = "TriggerSource" ("pFeatureName")
                  n242 = call "GetEnumFeatureEntryNum.vi"("pFeatureName"=w440, "handle"=w434, "error in (no error)"=w441) -> ("pEntryNum"=w433:i64, "error out"=w445:errorcluster)  [unwired: 7 in]
                  n243 = call "GetEnumFeatureEntrys.vi"("handle"=w434, "EntryNum"=w433, "pFeatureName"=w440, "error in (no error)"=w445) -> ("pLbEnumEntryList out"=w442:string, "error out"=w432:errorcluster)  [unwired: 5 in, 1 out]
                  n244 = for {
                    N: w433 -> [_]
                    shift-right: [w456] -> _
                    shift-left: 0 ("offset") -> [w457]
                    shift-right: [w454] -> _
                    shift-left: w442 -> [w455]
                    shift-right: [w452] -> w436
                    shift-left: string[] [] -> [w453]
                    n245 = Scan String For Tokens(6:string[] [":"] ("delimiters (\\s,\\t,\\r,\\n)"), 8:w457, 9:w455) -> (1:w451:string, 2:w456:i32, 3:w454:string)  [unwired: 3 in, 1 out]
                    n246 = Build Array (concatenate)(w453, w451) -> (w452:string[])
                  }
                  n247 = local read "handle"() -> (w438:i64)
                  n248 = property on="TriggerSource" class="Ring (strict)"(error in=w432, "Strings []"=w436) -> (error out=w439:errorcluster)  [unwired: 1 in, 1 out]
                  n249 = call "GetEnumFeatureSymbol.vi"("pFeatureName"="TriggerSource", "handle"=w438, "error in (no error)"=w439) -> ("pEnumSymbol"=w435:string, "error out"=w431:errorcluster)  [unwired: 7 in]
                  n250 = while {
                    tunnel: [w449] -> w430
                    tunnel: w436 -> [w448]
                    tunnel: w435 -> [w447]
                    i -> [w449]
                    stop <- w450 stop-if-true
                    n251 = Index Array(array=w448, index=w449) -> (element=w446:string)
                    n252 = Equal?(x=w446, y=w447) -> (x = y?=w450:bool)
                  }
                  n253 = property on="TriggerSource" class="Ring (strict)"(error in=w431, "Value"=w430) -> (error out=w429:errorcluster)  [unwired: 1 in, 1 out]
                }
              }
            }
            n254 = Merge Errors(w342) -> (w343:errorcluster)
          }
        }
      }
    }
    n255 = local read "QuitFlag"() -> (w325:bool)
    n256 = local write "error out"(w329) -> ()
  }
  n257 = while {
    tunnel: w1 -> [w461]
    stop <- w462 stop-if-true
    n258 = local read "IsGrabbing"() -> (w460:bool)
    n259 = case shown="True" w460 {
      tunnel: [w463 w467] -> w459
      tunnel: w461 -> [w463 w466]
      frame False {
      }
      frame True {
        n260 = local read "handle"() -> (w483:i64)
        n261 = call "GetFrame.vi"("timeoutMS"=500, "handle"=w483, "error in (no error)"=w466) -> ("frameHandle"=w465:i64, "pData"=w474:u8[], "pLbFrame out"=w475:T6, "error out"=w473:errorcluster, "return type"=w478:i32)  [unwired: 4 in]
        n262 = Equal To 0?(x=w478) -> (x = 0?=w477:bool)
        n263 = Unbundle By Name(w475) -> ("blockId"=w476:u64, "pixelFormat"=w471:i32)
        n264 = call <vilib>:"Calculate Frames per Second.vi"("Buffer Number"=w476) -> ("Processed Frames/s"=→"Processed Frames/s":dbl, "Acquired Frames/s"=→"Acquired Frames/s":dbl)  [unwired: 8 in, 1 out]
        n265 = case shown="True" w477 {
          tunnel: w475 -> [_ w504]
          tunnel: w474 -> [_ w508]
          tunnel: w473 -> [w486 w512]
          tunnel: [w486 w509] -> w472
          tunnel: w471 -> [_ w514]
          tunnel: w465 -> [w484 w506]
          tunnel: [w484 w506] -> w464
          frame False {
            n266 = Wait (ms)(milliseconds to wait=u32 2000 ("等待时间（毫秒）")) -> ()  [unwired: 1 out]
          }
          frame True {
            w491 = i16 0 ("left")
            n267 = Unbundle By Name(w504) -> ("width"=w496:u32, "height"=w503:u32, "size"=w502:u32, "pixelFormat"=w501:i32, "timeStamp"=w500:u64, "chunkCount"=w499:u32, "paddingX"=w498:u32, "paddingY"=w497:u32)
            n268 = local read "SavePic"() -> (w487:bool)
            n269 = property on="Picture" class="Pict"() -> ("Width"=w494:u32)  [unwired: 2 in, 2 out]
            n270 = case shown="17301505" w514 {
              tunnel: w508 -> [w542 w567]
              tunnel: [w547 w570] -> w518
              tunnel: [24 8] -> w519
              tunnel: [i32[] [] w576] -> w517
              tunnel: w512 -> [w546 w565]
              tunnel: [w550 w564] -> w511
              tunnel: [w542 w567] -> w507
              tunnel: [w535 w557] -> w505
              tunnel: w496 -> [w534 w554]
              tunnel: w503 -> [w533 w555]
              tunnel: w502 -> [w538 w561]
              tunnel: w501 -> [w539 w560]
              tunnel: w500 -> [_ _]
              tunnel: w499 -> [_ _]
              tunnel: w498 -> [w537 w559]
              tunnel: w497 -> [w536 w558]
              tunnel: [w534 w554] -> w493
              tunnel: [w534 w555] -> w489
              tunnel: [w533 w554] -> w488
              frame 0, Default {
                n271 = Compound Arithmetic op=MULTIPLY(u32 3 ("value"), w534, w533) -> (w535:u32)
                n272 = Bundle By Name(cluster="pConvertInfo In", "nWidth"=w534, "nHeight"=w533, "enSrcPixelType"=w539, "nSrcDataLen"=w538, "nPaddingX"=w537, "nPaddingY"=w536, "eBayerDemosaic"=u32 0, "eDstPixelFormat"=u32 35127316 ("enDstPixelType"), "nDstBufSize"=w535) -> (w543:T1)
                n273 = Initialize Array(u8 0, w535) -> (w544:u8[])
                n274 = local read "handle"() -> (w545:i64)
                n275 = call "PixelConvert.vi"("lbPstPixelConvertParam"=w543, "pDstBuf"=w544, "pSrcData"=w542, "handle"=w545, "error in (no error)"=w546) -> ("pDstBuf out"=w547:u8[], "error out"=w550:errorcluster)  [unwired: 4 in, 1 out]
              }
              frame 17301505 {
                n276 = Compound Arithmetic op=MULTIPLY(w554, w555, u32 3 ("value")) -> (w557:u32)
                n277 = for {
                  N: 256 -> [_]
                  shift-right: [w581] -> w576
                  shift-left: i32[] [] ("数组") -> [w580]
                  i -> [w577]
                  n278 = Subtract(x=255, y=w577) -> (x-y=w578:i32)
                  n279 = Logical Shift(y=i16 8, x=w578) -> (x << y=w583:i32)
                  n280 = Logical Shift(y=16 ("x"), x=w578) -> (x << y=w584:i32)
                  n281 = Compound Arithmetic op=ADD(w584, w583, w578) -> (w582:i32)
                  n282 = Build Array (concatenate)(w582, w580) -> (w581:i32[])
                }
                n283 = Bundle By Name(cluster="pConvertInfo In 2", "nWidth"=w554, "nHeight"=w555, "enSrcPixelType"=w560, "nSrcDataLen"=w561, "nPaddingX"=w559, "nPaddingY"=w558, "eBayerDemosaic"=u32 0, "eDstPixelFormat"=u32 17301505 ("enDstPixelType"), "nDstBufSize"=w557) -> (w568:T1)
                n284 = Initialize Array(u8 0, w557) -> (w571:u8[])
                n285 = local read "handle"() -> (w566:i64)
                n286 = call "PixelConvert.vi"("lbPstPixelConvertParam"=w568, "pDstBuf"=w571, "pSrcData"=w567, "handle"=w566, "error in (no error)"=w565) -> ("pDstBuf out"=w570:u8[], "error out"=w564:errorcluster)  [unwired: 4 in, 1 out]
              }
            }
            n287 = case shown="True" w487 {
              tunnel: w512 -> [w522 w532]
              tunnel: [w522 w531] -> w510
              tunnel: w504 -> [_ w528]
              tunnel: w507 -> [_ w524]
              tunnel: w505 -> [_ w523]
              frame False {
              }
              frame True {
                n288 = local read "Path"() -> (w526:path)
                n289 = Initialize Array(u8 0, w523) -> (w529:u8[])
                n290 = local read "handle"() -> (w527:i64)
                n291 = Path To String(path=w526) -> (string=w525:string)
                n292 = call "SaveImageToBmp.vi"("pSrcData"=w524, "handle"=w527, "pDstBuf"=w529, "fileName"=w525, "pLbFrame"=w528, "error in (no error)"=w532) -> ("error out"=w531:errorcluster)  [unwired: 4 in, 1 out]
              }
            }
            n293 = Divide(x=w494, y=w493) -> (x/y=w495:dbl)
            n294 = property on="Picture" class="Pict"("ZoomFactor"=w495) -> ()  [unwired: 2 in, 2 out]
            n295 = Bundle By Name(cluster="Rectangle", "left"=w491, "top"=w491, "right"=w489, "bottom"=w488) -> (w490:T3)
            n296 = Bundle By Name(cluster="image data", "image type"=0, "image depth"=w519, "image"=w518, "mask"=u8[] [], "colors"=w517, "Rectangle"=w490) -> (w513:T2)
            n297 = call <vilib>:"Draw Flattened Pixmap.vi"("image data"=w513) -> ("new picture"=→"Picture":picture)  [unwired: 8 in]
            n298 = Merge Errors(w510, w511) -> (w509:errorcluster)
          }
        }
        n299 = local read "handle"() -> (w479:i64)
        n300 = call "ReleaseFrame.vi"("frameHandle"=w464, "pData"=u8[] [1], "pLbFrame"=T5 {"blockId"=1, "status"=0, "width"=0, "height"=0, "size"=0, "pixelFormat"=0, "timeStamp"=0, "chunkCount"=0, "paddingX"=0, "paddingY"=0, "recvFrameTime"=0}, "handle"=w479, "error in (no error)"=w472) -> ("error out"=w467:errorcluster)  [unwired: 6 in]
        n301 = Wait (ms)(milliseconds to wait=u32 10 ("等待时间（毫秒）")) -> ()  [unwired: 1 out]
      }
    }
    n302 = local read "QuitFlag"() -> (w462:bool)
    n303 = local write "error out"(w459) -> ()
  }
